vi "datacluster_remove_zeros_speedmode.vi"(5 "reduce data pts":bool, 6 "# of final data pts":i32=5000, 7 "replace with interp. data":bool, 8 "iteration number":i32, 9 "remove zero":bool, 10 "Datasets to be processed":T1(array[cluster])=[{"String"="20120217.012", "Boolean"=TRUE, "begin"=15, "length"=10000, "y weight"=1.0}], 11 "data cluster":cluster{"all rows":dbl[][]}[](array[cluster])) -> (3 "data cluster out":cluster{"all rows":dbl[][]}[](array[cluster]))   [LabVIEW 2019]
panel:
  in  "start processing":bool
  in  "all columns":bool
  in  "target column":dbl
  # "Filter 1: Speed mode ON or OFF\nFileter 2: Remove Zero On or OFF\n    Replace with interp. data ON/OFF: When filter 2 is ON, the removed data were replaced by interpolated data"
  # "Caution: All rows will be affected."
  # "(1) Select datasets to be processed"
  # "(2) Reduce # of data if desired"
  # "(3) Select parameters for removing zeros"
  # "i) run zero-removing process?"
  # "ii) chose target column or perform for all columns"
  # "ii) after processing"
  # "delete data pts"
  # "(3) Start processing"
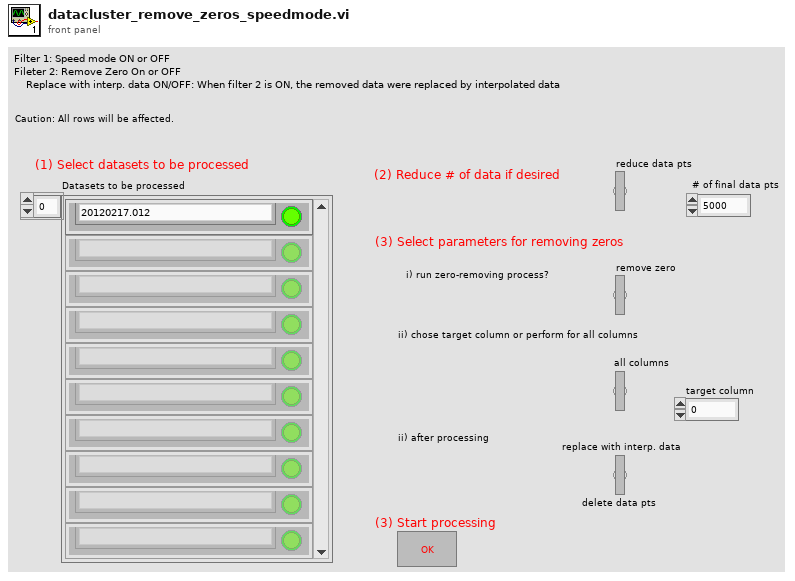
[diagram p1: front panel]
types:
  T1 = cluster{"String":string, "Boolean":bool, "begin":u32, "length":u32, "y weight":dbl}[]
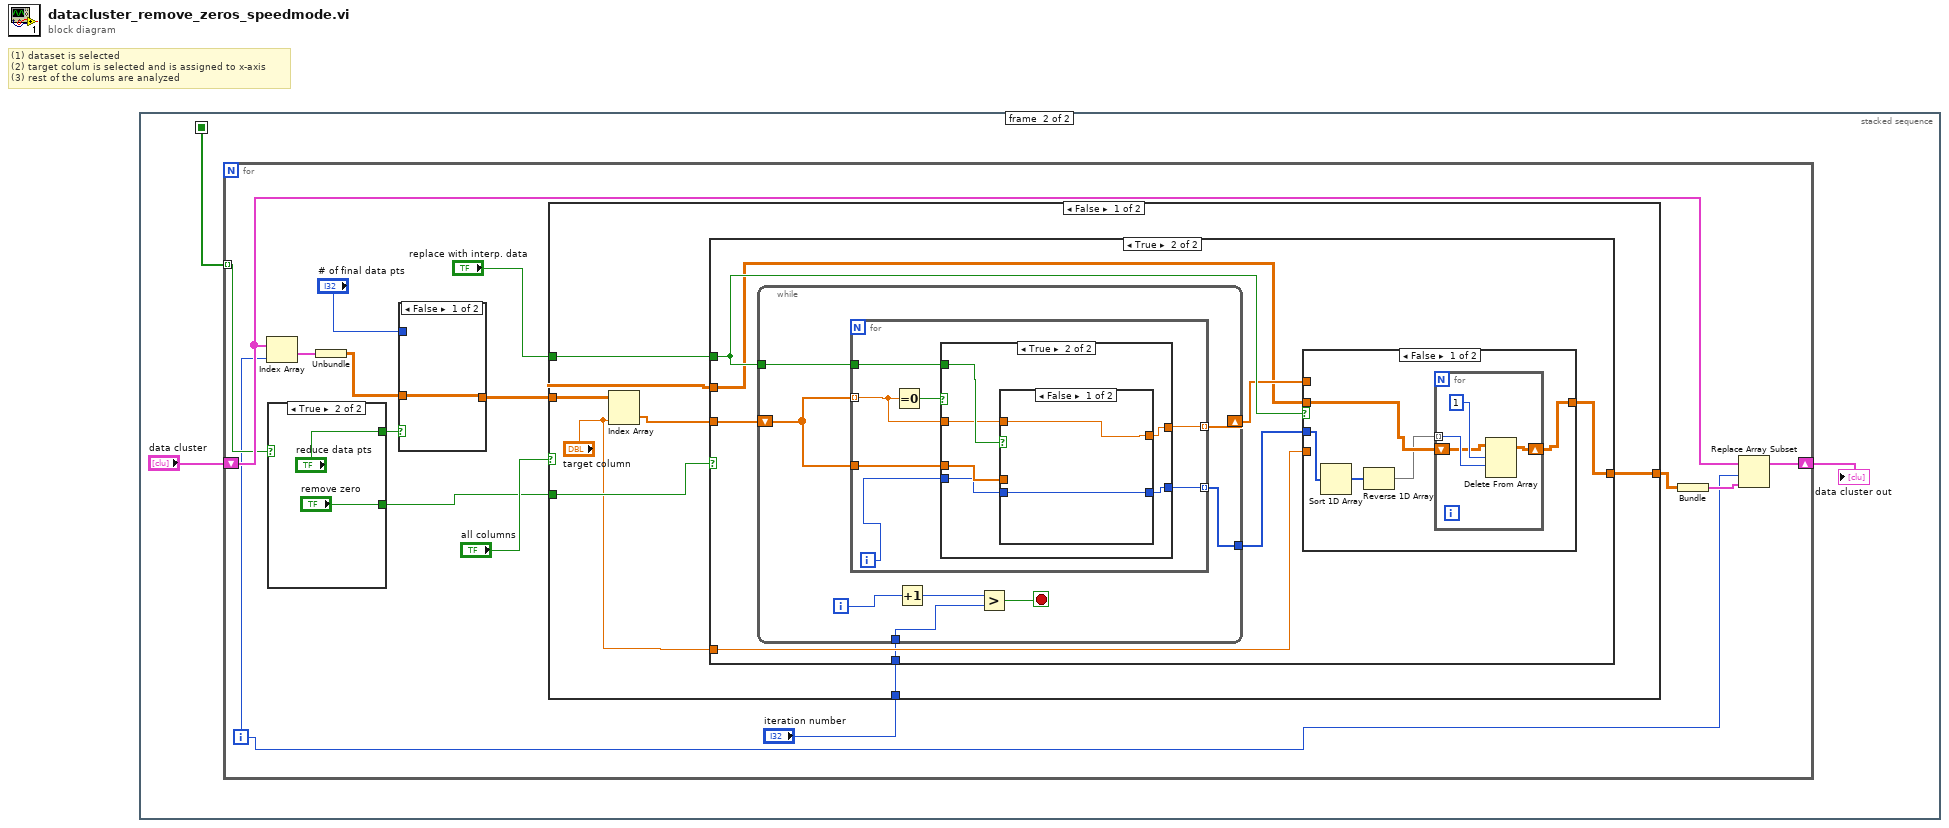
[diagram p0: block diagram]
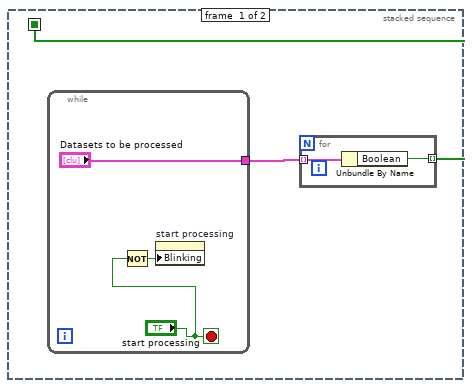
[diagram p2: hidden frame]
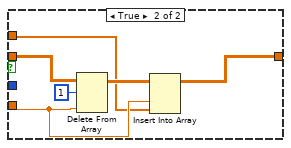
[diagram p5: hidden frame]
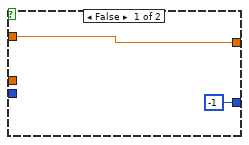
[diagram p6: hidden frame]
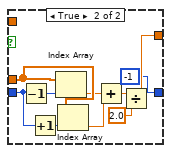
[diagram p7: hidden frame]
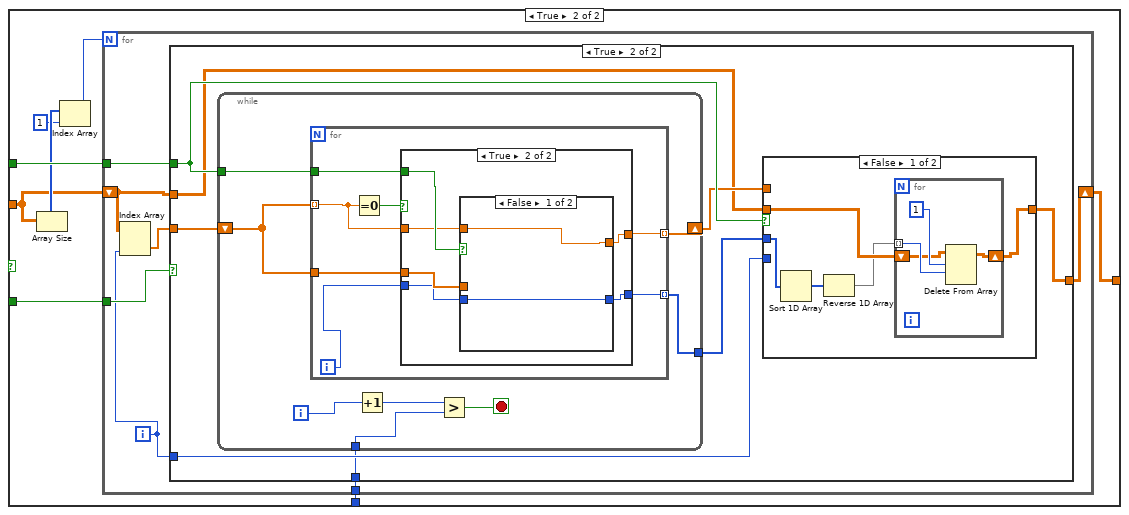
[diagram p8: hidden frame]
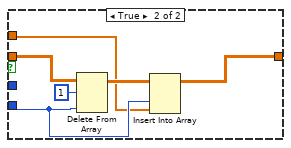
[diagram p10: hidden frame]
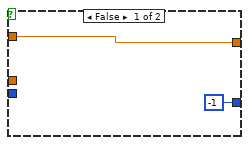
[diagram p11: hidden frame]
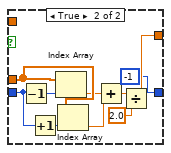
[diagram p12: hidden frame]
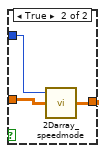
[diagram p13: hidden frame]
diagram:
  # "(1) dataset is selected\n(2) target colum is selected and is assigned to x-axis\n(3) rest of the colums are analyzed"
  n1 = stacked-sequence {
    seq-local: [w1 _] -> [_ w8]
    frame #0 {
      n2 = while {
        tunnel: ["Datasets to be processed"] -> w2
        stop <- "start processing" stop-if-true
        n3 = Not(x="start processing") -> (.not. x?=w6:bool)
        n4 = property on="start processing" class="Bool"("Blinking"=w6) -> ()  [unwired: 2 in, 2 out]
      }
      n5 = for {
        tunnel: w2 -> [w4] mode=indexing
        tunnel: [w3] -> w1 mode=indexing
        n6 = Unbundle By Name(w4) -> ("Boolean"=w3:bool)
      }
    }
    frame #1 {
      n7 = for {
        shift-right: [w14] -> w9
        shift-left: "data cluster" -> [w17]
        tunnel: w8 -> [w13] mode=indexing
        i -> [w11]
        n8 = Index Array(array=w17, index=w11) -> (element=w22:cluster{"all rows":dbl[][]})
        n9 = case shown="True" w13 {
          selector: w13 -> [w26 _]
          tunnel: [w26 "reduce data pts"] -> w25
          tunnel: [w26 "remove zero"] -> w12
          frame False {
          }
          frame True {
          }
        }
        n10 = Unbundle(w22) -> ("all rows"=w21:dbl[][])
        n11 = case shown="False" w25 {
          tunnel: [w169 w172] -> w20
          tunnel: "# of final data pts" -> [_ w171]
          tunnel: w21 -> [w169 w170]
          frame False {
          }
          frame True {
            n12 = call "2Darray_speedmode.vi"("original 2D array"=w170, "# of rows"=w171) -> ("reduced 2D array"=w172:dbl[][])  [unwired: 1 in]
          }
        }
        n13 = case shown="False" "all columns" {
          tunnel: w12 -> [w35 w102]
          tunnel: [w34 w99] -> w16
          tunnel: "replace with interp. data" -> [w33 w101]
          tunnel: w20 -> [w31 w95]
          tunnel: "iteration number" -> [w29 w100]
          frame False {
            n14 = Index Array(array=w31, index (col)="target column") -> (element=w32:dbl[])  [unwired: 1 in]
            n15 = case shown="True" w35 {
              tunnel: w32 -> [_ w44]
              tunnel: [w36 w41] -> w34
              tunnel: w33 -> [_ w43]
              tunnel: w31 -> [w36 w39]
              tunnel: "target column" -> [_ w38]
              tunnel: w29 -> [_ w37]
              frame False {
              }
              frame True {
                n16 = while {
                  shift-right: [w66] -> w42
                  shift-left: w44 -> [w67]
                  tunnel: w43 -> [w62]
                  tunnel: [w61] -> w40
                  tunnel: w37 -> [w60]
                  i -> [w65]
                  stop <- w64 stop-if-true
                  n17 = for {
                    tunnel: w67 -> [w73] mode=indexing
                    tunnel: [w74] -> w66 mode=indexing
                    tunnel: w67 -> [w72]
                    tunnel: w62 -> [w70]
                    tunnel: [w69] -> w61 mode=indexing
                    i -> [w71]
                    n18 = Equal To 0?(x=w73) -> (x = 0?=w68:bool)
                    n19 = case shown="True" w68 {
                      tunnel: [w76 w77] -> w74
                      tunnel: w73 -> [w76 w78]
                      tunnel: w72 -> [_ w82]
                      tunnel: w71 -> [_ w81]
                      tunnel: w70 -> [_ w80]
                      tunnel: [-1 w79] -> w69
                      frame False {
                      }
                      frame True {
                        n20 = case shown="False" w80 {
                          tunnel: w82 -> [_ w94]
                          tunnel: w81 -> [w84 w93]
                          tunnel: [w83 w86] -> w77
                          tunnel: [w84 -1] -> w79
                          tunnel: w78 -> [w83 _]
                          frame False {
                          }
                          frame True {
                            n21 = Decrement(x=w93) -> (x-1=w92:i32)
                            n22 = Increment(x=w93) -> (x+1=w91:i32)
                            n23 = Index Array(array=w94, index=w92) -> (element=w90:dbl)
                            n24 = Index Array(array=w94, index=w91) -> (element=w89:dbl)
                            n25 = Add(x=w90, y=w89) -> (x+y=w88:dbl)
                            n26 = Divide(x=w88, y=2.0) -> (x/y=w86:dbl)
                          }
                        }
                      }
                    }
                  }
                  n27 = Increment(x=w65) -> (x+1=w63:i32)
                  n28 = Greater?(x=w63, y=w60) -> (0:w64:bool)
                }
                n29 = case shown="False" w43 {
                  tunnel: w42 -> [_ w55]
                  tunnel: [w45 w54] -> w41
                  tunnel: w39 -> [w49 w59]
                  tunnel: w40 -> [w48 _]
                  tunnel: w38 -> [_ w56]
                  frame False {
                    n30 = Sort 1D Array(array=w48) -> (sorted array=w47:i32[])
                    n31 = Reverse 1D Array(array=w47) -> (reversed array=w46:i32[])
                    n32 = for {
                      tunnel: w46 -> [w53] mode=indexing
                      shift-right: [w50] -> w45
                      shift-left: w49 -> [w51]
                      n33 = Delete From Array(array=w51, length=1, index (row)=w53) -> (array with subset deleted=w50:dbl[][])  [unwired: 1 in, 1 out]
                    }
                  }
                  frame True {
                    n34 = Delete From Array(array=w59, length=1, index (col)=w56) -> (array with subset deleted=w57:dbl[][])  [unwired: 1 in, 1 out]
                    n35 = Insert Into Array(array=w57, index (col)=w56, new element=w55) -> (w54:dbl[][])  [unwired: 1 in]
                  }
                }
              }
            }
          }
          frame True {
            n36 = Array Size(array=w95) -> (size(s)=w98:i32[])
            n37 = Index Array(array=w98, index=1) -> (element=w96:i32)
            n38 = for {
              N: w96 -> [_]
              tunnel: w102 -> [w109]
              tunnel: w101 -> [w108]
              tunnel: w100 -> [w107]
              shift-right: [w106] -> w99
              shift-left: w95 -> [w103]
              i -> [w104]
              n39 = Index Array(array=w103, index (col)=w104) -> (element=w105:dbl[])  [unwired: 1 in]
              n40 = case shown="True" w109 {
                tunnel: w105 -> [_ w118]
                tunnel: [w110 w115] -> w106
                tunnel: w108 -> [_ w117]
                tunnel: w103 -> [w110 w113]
                tunnel: w104 -> [_ w112]
                tunnel: w107 -> [_ w111]
                frame False {
                }
                frame True {
                  n41 = while {
                    shift-right: [w140] -> w116
                    shift-left: w118 -> [w141]
                    tunnel: w117 -> [w136]
                    tunnel: [w135] -> w114
                    tunnel: w111 -> [w134]
                    i -> [w139]
                    stop <- w138 stop-if-true
                    n42 = for {
                      tunnel: w141 -> [w147] mode=indexing
                      tunnel: [w148] -> w140 mode=indexing
                      tunnel: w141 -> [w146]
                      tunnel: w136 -> [w144]
                      tunnel: [w143] -> w135 mode=indexing
                      i -> [w145]
                      n43 = Equal To 0?(x=w147) -> (x = 0?=w142:bool)
                      n44 = case shown="True" w142 {
                        tunnel: [w150 w151] -> w148
                        tunnel: w147 -> [w150 w152]
                        tunnel: w146 -> [_ w156]
                        tunnel: w145 -> [_ w155]
                        tunnel: w144 -> [_ w154]
                        tunnel: [-1 w153] -> w143
                        frame False {
                        }
                        frame True {
                          n45 = case shown="False" w154 {
                            tunnel: w156 -> [_ w168]
                            tunnel: w155 -> [w158 w167]
                            tunnel: [w157 w160] -> w151
                            tunnel: [w158 -1] -> w153
                            tunnel: w152 -> [w157 _]
                            frame False {
                            }
                            frame True {
                              n46 = Decrement(x=w167) -> (x-1=w166:i32)
                              n47 = Increment(x=w167) -> (x+1=w165:i32)
                              n48 = Index Array(array=w168, index=w166) -> (element=w164:dbl)
                              n49 = Index Array(array=w168, index=w165) -> (element=w163:dbl)
                              n50 = Add(x=w164, y=w163) -> (x+y=w162:dbl)
                              n51 = Divide(x=w162, y=2.0) -> (x/y=w160:dbl)
                            }
                          }
                        }
                      }
                    }
                    n52 = Increment(x=w139) -> (x+1=w137:i32)
                    n53 = Greater?(x=w137, y=w134) -> (0:w138:bool)
                  }
                  n54 = case shown="False" w117 {
                    tunnel: w116 -> [_ w129]
                    tunnel: [w119 w128] -> w115
                    tunnel: w113 -> [w123 w133]
                    tunnel: w114 -> [w122 _]
                    tunnel: w112 -> [_ w130]
                    frame False {
                      n55 = Sort 1D Array(array=w122) -> (sorted array=w121:i32[])
                      n56 = Reverse 1D Array(array=w121) -> (reversed array=w120:i32[])
                      n57 = for {
                        tunnel: w120 -> [w127] mode=indexing
                        shift-right: [w124] -> w119
                        shift-left: w123 -> [w125]
                        n58 = Delete From Array(array=w125, length=1, index (row)=w127) -> (array with subset deleted=w124:dbl[][])  [unwired: 1 in, 1 out]
                      }
                    }
                    frame True {
                      n59 = Delete From Array(array=w133, length=1, index (col)=w130) -> (array with subset deleted=w131:dbl[][])  [unwired: 1 in, 1 out]
                      n60 = Insert Into Array(array=w131, index (col)=w130, new element=w129) -> (w128:dbl[][])  [unwired: 1 in]
                    }
                  }
                }
              }
            }
          }
        }
        n61 = Bundle("reduced 2D array"=w16) -> (w15:cluster{"reduced 2D array":dbl[][]})  [unwired: 1 in]
        n62 = Replace Array Subset(array=w17, new element=w15, index=w11) -> (w14:cluster{"all rows":dbl[][]}[])
      }
      "data cluster out" <- w9
    }
  }
